vi "IN Stack Weigh-RS232-SendandReceiveMessage.vi"(8 "错误输入（无错误）":errorcluster, 9 "CommandZERO":string="*IDN?\n", 10 "Command":string="*IDN?\n", 11 "VISA资源名称":refnum<visa-resource-name>) -> (0 "错误输出":errorcluster, 1 "响应":string, 2 "异常结果":bool, 3 "VISA资源名称输出":refnum<visa-resource-name>)   [LabVIEW 2015]
uses:
  <vilib>/Instr/_visa.llb/VISA Flush IO Buffer Mask.ctl
  C:/Program Files (x86)/National Instruments/LabVIEW 2015/examples/Instrument IO/Serial/support/Serial - Settings.ctl
  <vilib>/Instr/_visa.llb/VISA Configure Serial Port (Instr).vi
panel:
  out "read buffer":string
  in  "读取前延时(ms)":u32=300
  out "读取的字节":u32
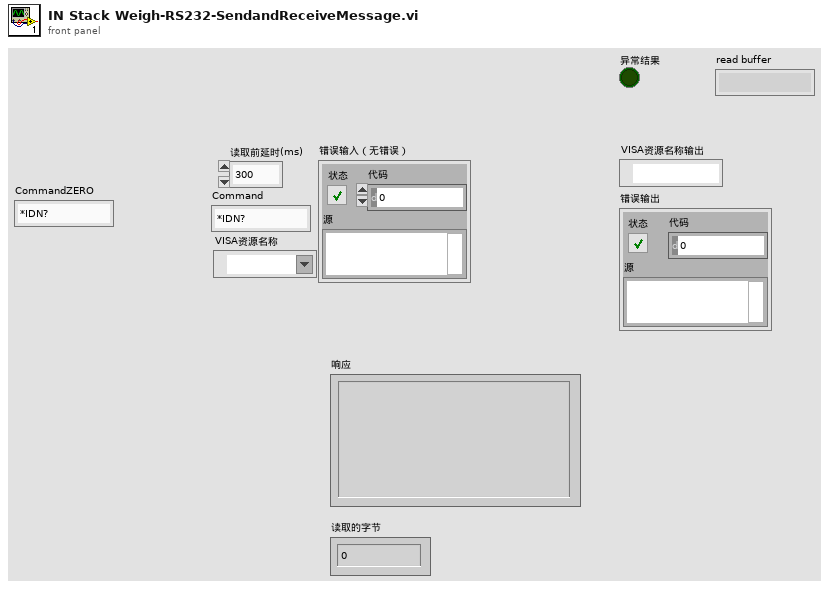
[diagram p1: front panel]
types:
  T1 = typedef "VISA Flush IO Buffer Mask.ctl" = u16
  T2 = typedef "Serial - Settings.ctl" = cluster{"波特率":u32, "数据比特":u16, "奇偶":enum16{"None", "Odd", "Even", "Mark", "Space"}, "停止位":u16, "流控制":u16}
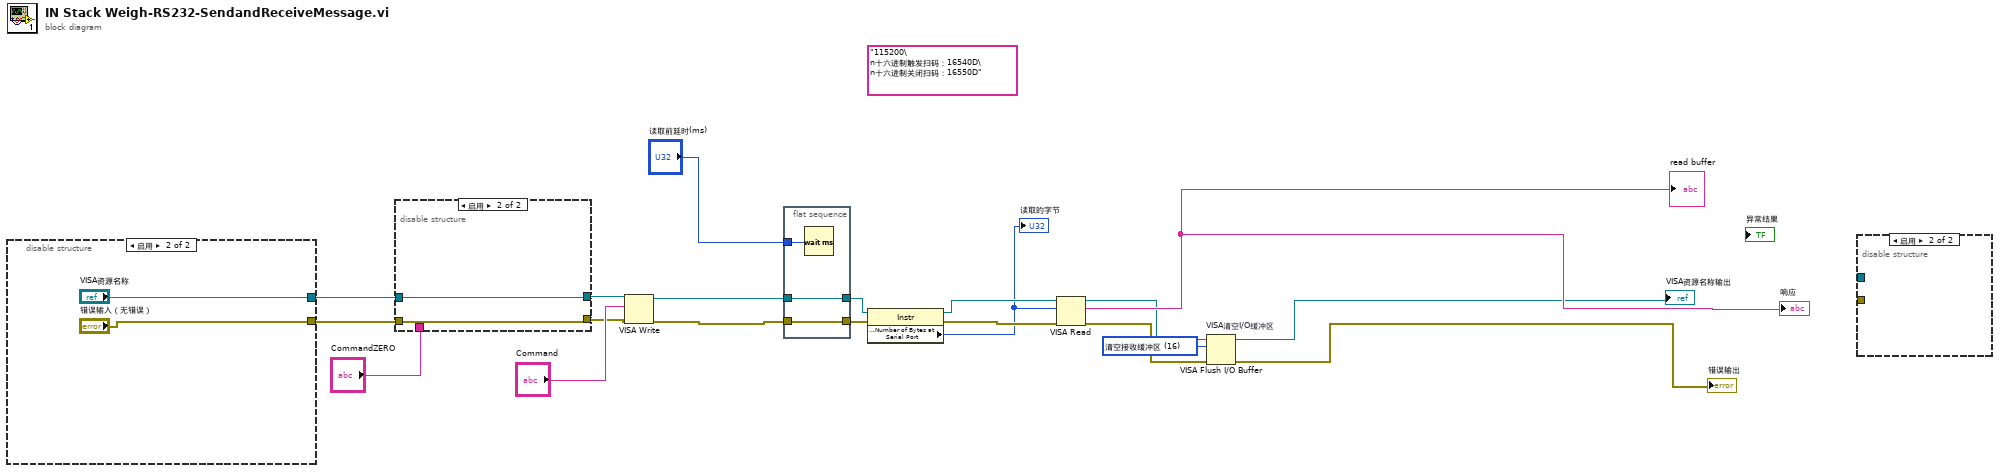
[diagram p0: block diagram]
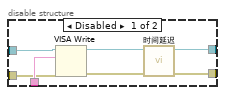
[diagram p2: hidden frame]
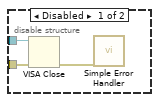
[diagram p3: hidden frame]
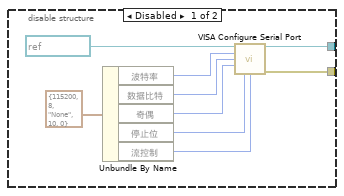
[diagram p4: hidden frame]
diagram:
  w1 = T1 16 items=["清空接收缓冲区"=16, "向设备写入传输缓冲区"=32, "清空接收缓冲区（无I/O）"=64, "清空传输缓冲区"=128] ("Mask")
  (unwired) "115200\n十六进制触发扫码：16540D\n十六进制关闭扫码：16550D"
  n1 = disable-structure shown="启用" {
    disable-tunnel: [w22 "VISA资源名称"] -> w9
    disable-tunnel: [w21 "错误输入（无错误）"] -> w8
    frame Disabled {
      n2 = Unbundle By Name(T2 {"波特率"=115200, "数据比特"=8, "奇偶"=enum."None", "停止位"=10, "流控制"=0} ("串口设置")) -> ("波特率"=w29:u32, "数据比特"=w28:u16, "奇偶"=w27:enum16{"None", "Odd", "Even", "Mark", "Space"}, "停止位"=w26:u16, "流控制"=w25:u16)
      n3 = call-poly "VISA Configure Serial Port"("VISA resource name"=refnum<visa-resource-name> "COM5" ("VISA资源名称"), "baud rate (9600)"=w29, "data bits (8)"=w28, "parity (0:none)"=w27, "stop bits (10: 1 bit)"=w26, "flow control (0:none)"=w25) -> ("VISA resource name out"=w22:refnum<visa-resource-name>, "error out"=w21:errorcluster)  [unwired: 3 in, 5 out]
    }
    frame Enabled {
    }
  }
  n4 = disable-structure shown="启用" {
    disable-tunnel: "CommandZERO" -> [w37 _]
    disable-tunnel: w9 -> [w36 w39]
    disable-tunnel: w8 -> [w35 w38]
    disable-tunnel: [w34 w39] -> w7
    disable-tunnel: [w32 w38] -> w6
    frame Disabled {
      n5 = VISA Write(VISA resource name=w36, write buffer=w37, error in (no error)=w35) -> (VISA resource name out=w34:refnum<visa-resource-name>, error out=w33:errorcluster)  [unwired: 1 out]
      n6 = call "时间延迟"("error in (no error)"=w33) -> ("error out"=w32:errorcluster)  [unwired: 10 in]
    }
    frame Enabled {
    }
  }
  n7 = VISA Write(VISA resource name=w7, write buffer="Command", error in (no error)=w6) -> (VISA resource name out=w19:refnum<visa-resource-name>, error out=w20:errorcluster)  [unwired: 1 out]
  n8 = flat-sequence {
    tunnel: w20 -> [w41]
    tunnel: [w41] -> w15
    tunnel: w19 -> [w40]
    tunnel: [w40] -> w14
    tunnel: "读取前延时(ms)" -> [w42]
    frame #0 {
      n9 = Wait (ms)(milliseconds to wait=w42) -> ()  [unwired: 1 out]
    }
  }
  n10 = property class="Instr"(reference=w14, error in=w15) -> (reference out=w13:refnum<visa-resource-name>, error out=w12:errorcluster, "Serial Settings:Number of Bytes at Serial Port"=w11:u32)
  "读取的字节" <- w11
  n11 = VISA Read(VISA resource name=w13, byte count=w11, error in (no error)=w12) -> (VISA resource name out=w5:refnum<visa-resource-name>, read buffer=→"响应" →"read buffer":string, error out=w3:errorcluster)  [unwired: 1 out]
  n12 = VISA Flush I/O Buffer "VISA清空I/O缓冲区"(VISA resource name=w5, mask (16)=w1, error in (no error)=w3) -> (VISA resource name out=→"VISA资源名称输出":refnum<visa-resource-name>, error out=→"错误输出":errorcluster)
  n13 = disable-structure shown="启用" {
    disable-tunnel: _ -> [w44 _]
    disable-tunnel: _ -> [w43 _]
    frame Disabled {
      n14 = VISA Close(VISA resource name=w44, error in (no error)=w43) -> (error out=w45:errorcluster)
      n15 = call <vilib>:"Simple Error Handler.vi"("error in (no error)"=w45) -> ()  [unwired: 1 in, 8 out]
    }
    frame Enabled {
    }
  }
